vi "Get Supported Targets.vi"(8 "error in":errorcluster, 11 "Scan Engine configuration in":refnum<class "Scan Engine configuration.lvclass">) -> (0 "error out":errorcluster, 2 "supported targets":T1[](array[typedef]), 3 "Scan Engine configuration out":refnum<class "Scan Engine configuration.lvclass">)   [LabVIEW 2013, in "Scan Engine configuration.lvclass"]
doc: "Provides an interface for determining the targets supported by a given module configuration/runtime class pairing. This should be overridden by any useful child class."
uses:
  Scan Engine configuration.lvclass
  <vilib>/NI/Tag Bus Module Framework/root configuration/Target Types.ctl
  <vilib>/NI/Tag Bus Module Framework/root configuration/TBM configuration.lvclass
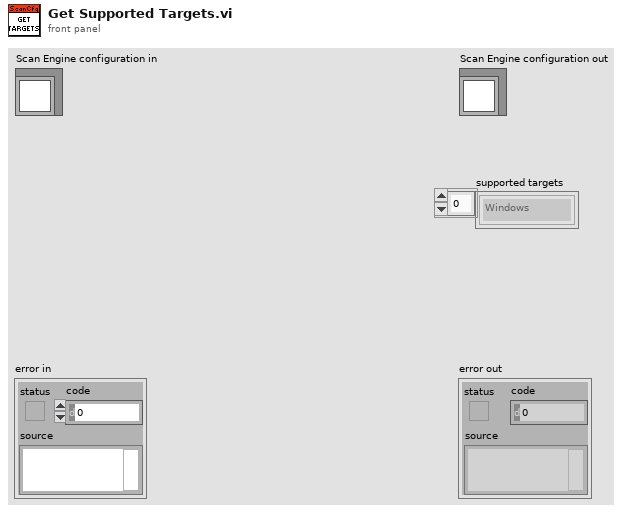
[diagram p1: front panel]
types:
  T1 = typedef "TBM configuration.lvclass/Target Types.ctl" = enum16{"Windows", "Mac", "Linux", "Linux RT ARM", "VxWorks", "Pharlap", "Other", "Linux RT x64"}
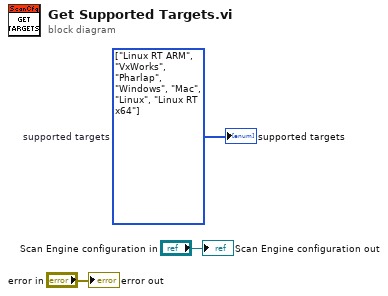
[diagram p0: block diagram]
diagram:
  w1 = T1[] [enum."Linux RT ARM", enum."VxWorks", enum."Pharlap", enum."Windows", enum."Mac", enum."Linux", enum."Linux RT x64"] items=["Windows", "Mac", "Linux", "Linux RT ARM", "VxWorks", "Pharlap", "Other", "Linux RT x64"]  # supported targets
  "error out" <- "error in"
  "Scan Engine configuration out" <- "Scan Engine configuration in"
  "supported targets" <- w1
